vi "interface_select_class.vi"(8 "error in (no error)":errorcluster) -> (0 "error out":errorcluster, 3 "builder_class file":path)   [LabVIEW 2015, in "lv-build-interface.lvlib"]
uses:
  lv-build-interface.lvlib
  <vilib>/Utility/error.llb/Error Cluster From Error Code.vi
  <vilib>/ErrorRing/Error Ring.xnode
  lv-builder/lv-builder.lvlib
panel:
  in  "refresh":bool
  in  "select_class":bool
  in  "tree":i32(listbox)
  in  "open_class":bool
  in  "cancel":bool
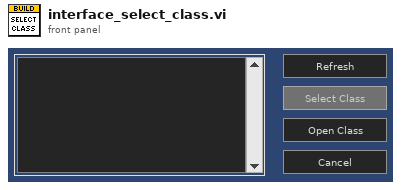
[diagram p1: front panel]
types:
  T1 = enum8{"Enabled", "Disabled", "Disabled and Grayed Out"}
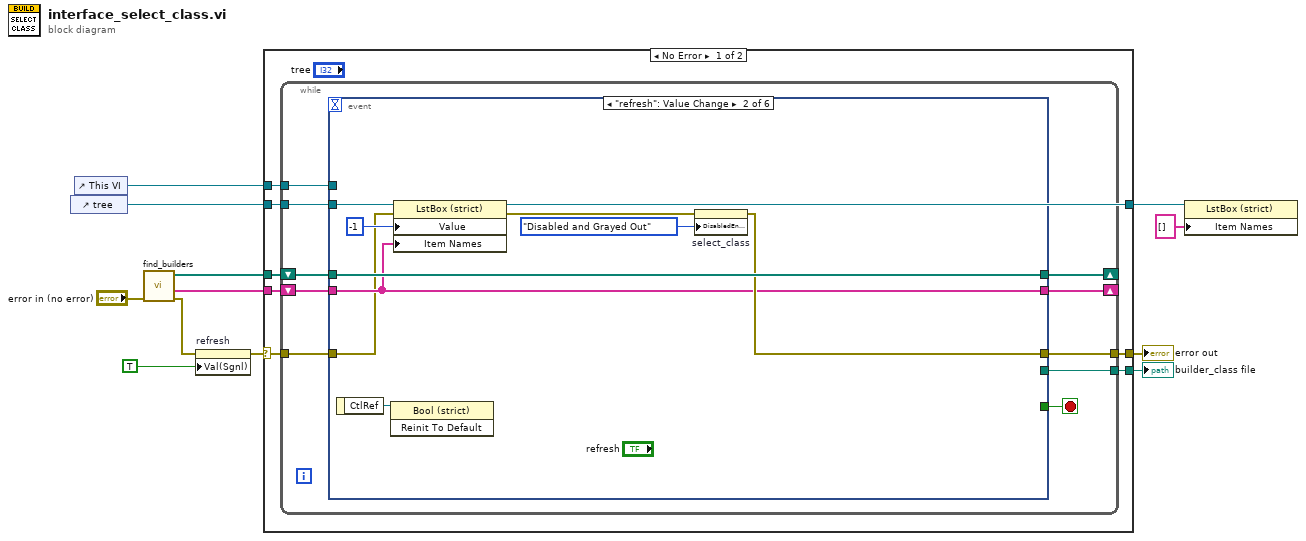
[diagram p0: block diagram]
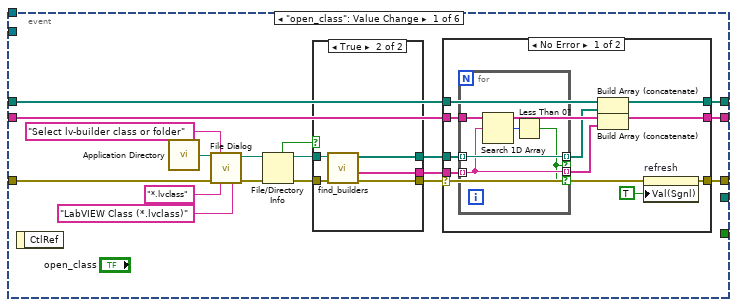
[diagram p2: hidden frame]
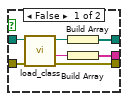
[diagram p3: hidden frame]
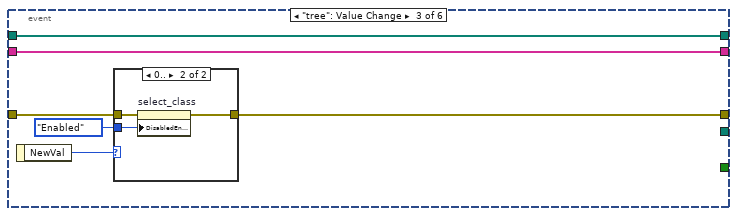
[diagram p5: hidden frame]
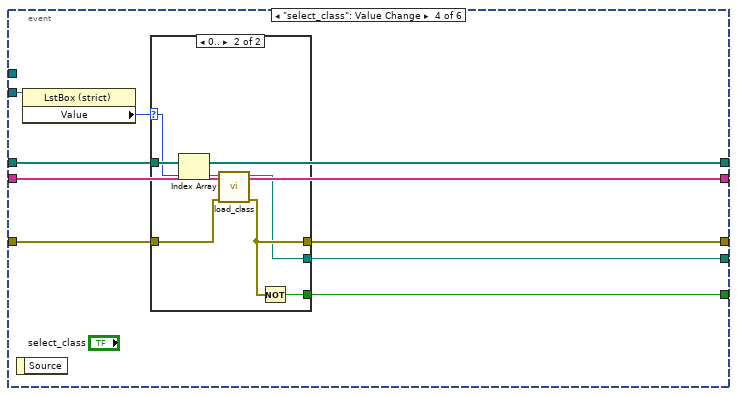
[diagram p7: hidden frame]
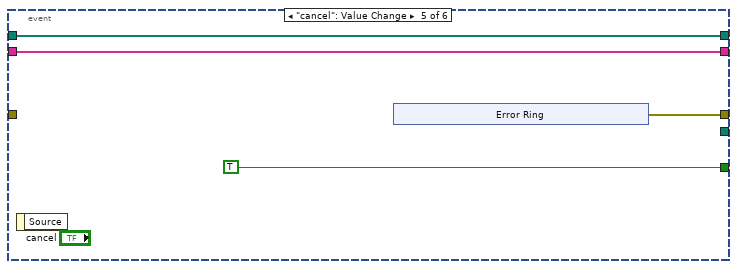
[diagram p9: hidden frame]
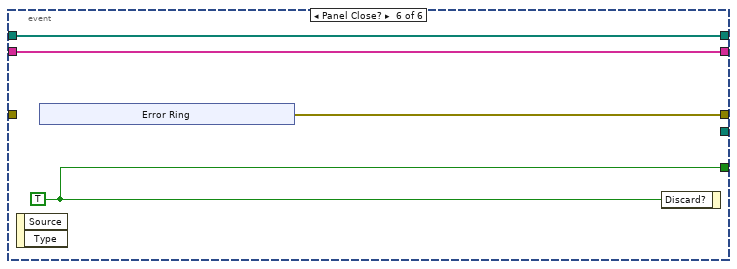
[diagram p10: hidden frame]
diagram:
  n1 = control-ref of="tree"() -> (w12:refnum<vi>)
  n2 = control-ref of="This VI"() -> (w9:refnum<vi>)
  n3 = call "find_builders.vi"("error in (no error)"="error in (no error)") -> ("error out"=w3:errorcluster, "name []"=w1:string[], "path []"=w2:path[])  [unwired: 7 in, 1 out]
  n4 = property on="refresh" class="Bool (strict)"(error in=w3, "Val(Sgnl)"=TRUE ("Value (Signaling)")) -> (error out=w7:errorcluster)  [unwired: 1 in, 1 out]
  n5 = case shown="No Error" w7 {
    selector: w7 -> [w17 w131]
    tunnel: [w19 w131] -> w8
    tunnel: w9 -> [w18 _]
    tunnel: w12 -> [w15 w130]
    tunnel: w2 -> [w16 _]
    tunnel: [w15 w130] -> w11
    tunnel: w1 -> [w14 _]
    tunnel: [w13 _] -> w5
    frame No Error {
      n6 = while {
        tunnel: [w21] -> w19
        tunnel: w17 -> [w29]
        tunnel: w18 -> [w25]
        tunnel: w15 -> [w28]
        shift-right: [w24] -> _
        shift-left: w16 -> [w26]
        shift-right: [w22] -> _
        shift-left: w14 -> [w23]
        tunnel: [w20] -> w13
        stop <- w27 stop-if-true
        n7 = event shown="[1] \"refresh\": Value Change" {
          selector: _ -> [_ _ _ _ _ _]
          dyn-events: _ -> [_ _ _ _ _ _]
          timeout: _ -> [_ _ _ _ _ _]
          tunnel: [w44 w81 w90 w100 w116 w122] -> w21
          tunnel: w29 -> [w45 w79 w91 w102 _ _]
          tunnel: w25 -> [_ _ _ _ _ _]
          tunnel: w28 -> [_ w83 _ w105 _ _]
          tunnel: [_ _ _ w101 TRUE w125] -> w27
          tunnel: w26 -> [w47 w87 w88 w103 w114 w123]
          tunnel: [w46 w87 w88 w103 w114 w123] -> w24
          tunnel: [w30 w80 w89 w99 w115 w124] -> w22
          tunnel: w23 -> [w31 w80 w89 w99 w115 w124]
          tunnel: [_ _ _ w98 _ _] -> w20
          event "open_class": Value Change {
            n8 = event-data() -> ()  [unwired: 1 in, 1 out]
            n9 = call <vilib>:"Application Directory.vi"() -> ("Application Directory"=w42:path)
            n10 = call "File Dialog"("start path"=w42, "prompt"="Select lv-builder class or folder", "error in"=w45, "pattern (all files)"="*.lvclass" ("filter"), "pattern label"="LabVIEW Class (*.lvclass)" ("filter")) -> ("selected path"=w38:path, "error out"=w37:errorcluster)  [unwired: 7 in, 2 out]
            n11 = File/Directory Info(path=w38, error in=w37) -> (path out=w33:path, directory=w34:bool, error out=w35:errorcluster)  [unwired: 4 out]
            n12 = case shown="True" w34 {
              tunnel: [w53 w57] -> w39
              tunnel: [w48 w56] -> w36
              tunnel: w35 -> [w54 w59]
              tunnel: w33 -> [w52 w58]
              tunnel: [w49 w55] -> w32
              frame False {
                n13 = call "load_class.vi"("error in (no error)"=w54, "builder_class in"=w52) -> ("error out"=w53:errorcluster, "name"=w50:string, "builder_class out"=w51:path)  [unwired: 6 in, 1 out]
                n14 = Build Array(w51) -> (w48:path[])
                n15 = Build Array(w50) -> (w49:string[])
              }
              frame True {
                n16 = call "find_builders.vi"("error in (no error)"=w59, "folder"=w58) -> ("error out"=w57:errorcluster, "name []"=w55:string[], "path []"=w56:path[])  [unwired: 6 in, 1 out]
              }
            }
            n17 = case shown="No Error" w39 {
              selector: w39 -> [w66 w78]
              tunnel: w36 -> [w64 _]
              tunnel: [w65 w78] -> w44
              tunnel: w47 -> [w70 w77]
              tunnel: [w69 w77] -> w46
              tunnel: w32 -> [w63 _]
              tunnel: w31 -> [w62 w76]
              tunnel: [w68 w76] -> w30
              frame No Error {
                n18 = for {
                  tunnel: w64 -> [w74] mode=indexing
                  tunnel: w63 -> [w73] mode=indexing
                  tunnel: w62 -> [w75]
                  tunnel: [w74] -> w61 mode=indexing if=w71
                  tunnel: [w73] -> w60 mode=indexing if=w71
                  n19 = Search 1D Array(1D array=w75, element=w73) -> (index of element=w72:i32)  [unwired: 1 in]
                  n20 = Less Than 0?(x=w72) -> (x < 0?=w71:bool)
                }
                n21 = Build Array (concatenate)(w70, w61) -> (w69:path[])
                n22 = Build Array (concatenate)(w62, w60) -> (w68:string[])
                n23 = property on="refresh" class="Bool (strict)"(error in=w66, "Val(Sgnl)"=TRUE ("Value (Signaling)")) -> (error out=w65:errorcluster)  [unwired: 1 in, 1 out]
              }
              frame Error {
              }
            }
          }
          event "refresh": Value Change {
            n24 = event-data() -> ("CtlRef"=w82:refnum<vi>)  [unwired: 1 in]
            n25 = invoke class="Bool (strict)" method="Reinit To Default"(reference=w82) -> ()  [unwired: 2 in, 3 out]
            n26 = property class="LstBox (strict)"(reference=w83, error in=w79, "Value"=-1, "Item Names"=w80) -> (error out=w85:errorcluster)  [unwired: 1 out]
            n27 = property on="select_class" class="Bool"(error in=w85, "DisabledEnum"=T1."Disabled and Grayed Out" ("Disabled")) -> (error out=w81:errorcluster)  [unwired: 1 in, 1 out]
          }
          event "tree": Value Change {
            n28 = event-data() -> ("NewVal"=w92:i32)  [unwired: 1 in]
            n29 = case shown="0.." w92 {
              tunnel: T1."Enabled" ("Disabled") -> [_ w97]
              tunnel: w91 -> [w94 w96]
              tunnel: [w94 w95] -> w90
              frame Default {
              }
              frame 0.. {
                n30 = property on="select_class" class="Bool"(error in=w96, "DisabledEnum"=w97) -> (error out=w95:errorcluster)  [unwired: 1 in, 1 out]
              }
            }
          }
          event "select_class": Value Change {
            n31 = event-data() -> ()  [unwired: 1 in, 1 out]
            n32 = property class="LstBox (strict)"(reference=w105) -> ("Value"=w104:i32)  [unwired: 1 in, 2 out]
            n33 = case shown="0.." w104 {
              selector: w104 -> [_ w111]
              tunnel: w103 -> [_ w112]
              tunnel: w102 -> [w106 w113]
              tunnel: [_ w109] -> w101
              tunnel: [w106 w108] -> w100
              tunnel: [_ w107] -> w98
              frame Default {
              }
              frame 0.. {
                n34 = Index Array(array=w112, index=w111) -> (element=w110:path)
                n35 = call "load_class.vi"("error in (no error)"=w113, "builder_class in"=w110) -> ("error out"=w108:errorcluster, "builder_class out"=w107:path)  [unwired: 6 in, 2 out]
                n36 = Not(x=w108) -> (.not. x?=w109:bool)
              }
            }
          }
          event "cancel": Value Change {
            n37 = event-data() -> ()  [unwired: 1 in, 1 out]
            n38 = xnode "Error Ring"() -> ("error out"=w116:errorcluster)
          }
          event Panel Close? {
            w125 = TRUE
            n39 = event-data() -> ()  [unwired: 1 in, 2 out]
            n40 = xnode "Error Ring"() -> ("error out"=w122:errorcluster)
            n41 = event-data("Discard?"=w125) -> ()  [unwired: 1 in, 1 out]
          }
        }
      }
    }
    frame Error {
    }
  }
  "error out" <- w8
  "builder_class file" <- w5
  n42 = property class="LstBox (strict)"(reference=w11, "Item Names"=string[] []) -> ()  [unwired: 1 in, 2 out]
